vi "AddBall.vi"(8 "Boolean":bool, 9 "Numeric":dbl, 10 "Array":u32[][](array[numeric]), 11 "Refnum in":T1) -> (3 "Refnum out":T1)   [LabVIEW 2018]
uses:
  <vilib>/vision/Image Controls.llb/IMAQ Image.ctl
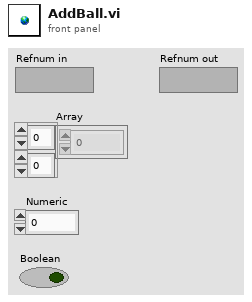
[diagram p1: front panel]
types:
  T1 = typedef "IMAQ Image.ctl" = refnum<image>
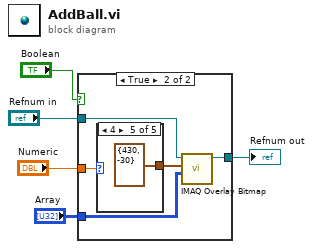
[diagram p0: block diagram]
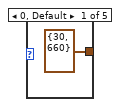
[diagram p3: hidden frame]
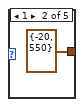
[diagram p4: hidden frame]
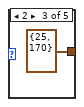
[diagram p5: hidden frame]
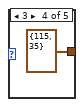
[diagram p6: hidden frame]
diagram:
  n1 = case shown="True" "Boolean" {
    tunnel: "Refnum in" -> [w6 w11]
    tunnel: [w6 w10] -> w5
    tunnel: "Numeric" -> [_ w9]
    tunnel: "Array" -> [_ w7]
    frame False {
    }
    frame True {
      n2 = case shown="4" w9 {
        tunnel: [cluster{"X":i32, "Y":i32} {"X"=30, "Y"=660} ("Top Left Point") cluster{"X":i32, "Y":i32} {"X"=-20, "Y"=550} ("Top Left Point") cluster{"X":i32, "Y":i32} {"X"=25, "Y"=170} ("Top Left Point") cluster{"X":i32, "Y":i32} {"X"=115, "Y"=35} ("Top Left Point") cluster{"X":i32, "Y":i32} {"X"=430, "Y"=-30} ("Top Left Point")] -> w8
        frame 0, Default {
        }
        frame 1 {
        }
        frame 2 {
        }
        frame 3 {
        }
        frame 4 {
        }
      }
      n3 = call "IMAQ Overlay Bitmap"("Bitmap"=w7, "Top Left Point"=w8, "Image"=w11) -> ("Image Out"=w10:T1)  [unwired: 7 in, 1 out]
    }
  }
  "Refnum out" <- w5
